vi "反控数据上传(子VI).vi"(8 "error in (no error)":errorcluster caption="错误输入（无错误）", 11 "QN":string) -> (0 "error out":errorcluster caption="错误输出")   [LabVIEW 2016, in "数据传输系统.lvlib"]
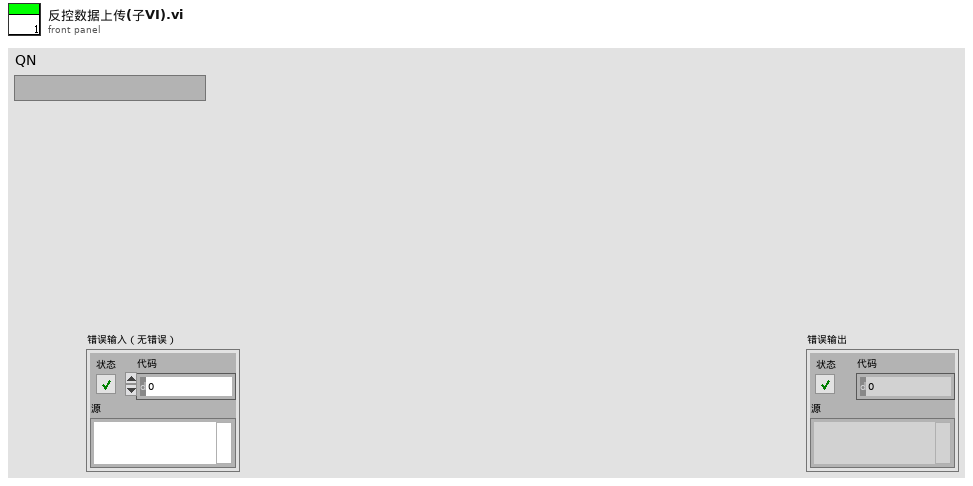
[diagram p1: front panel]
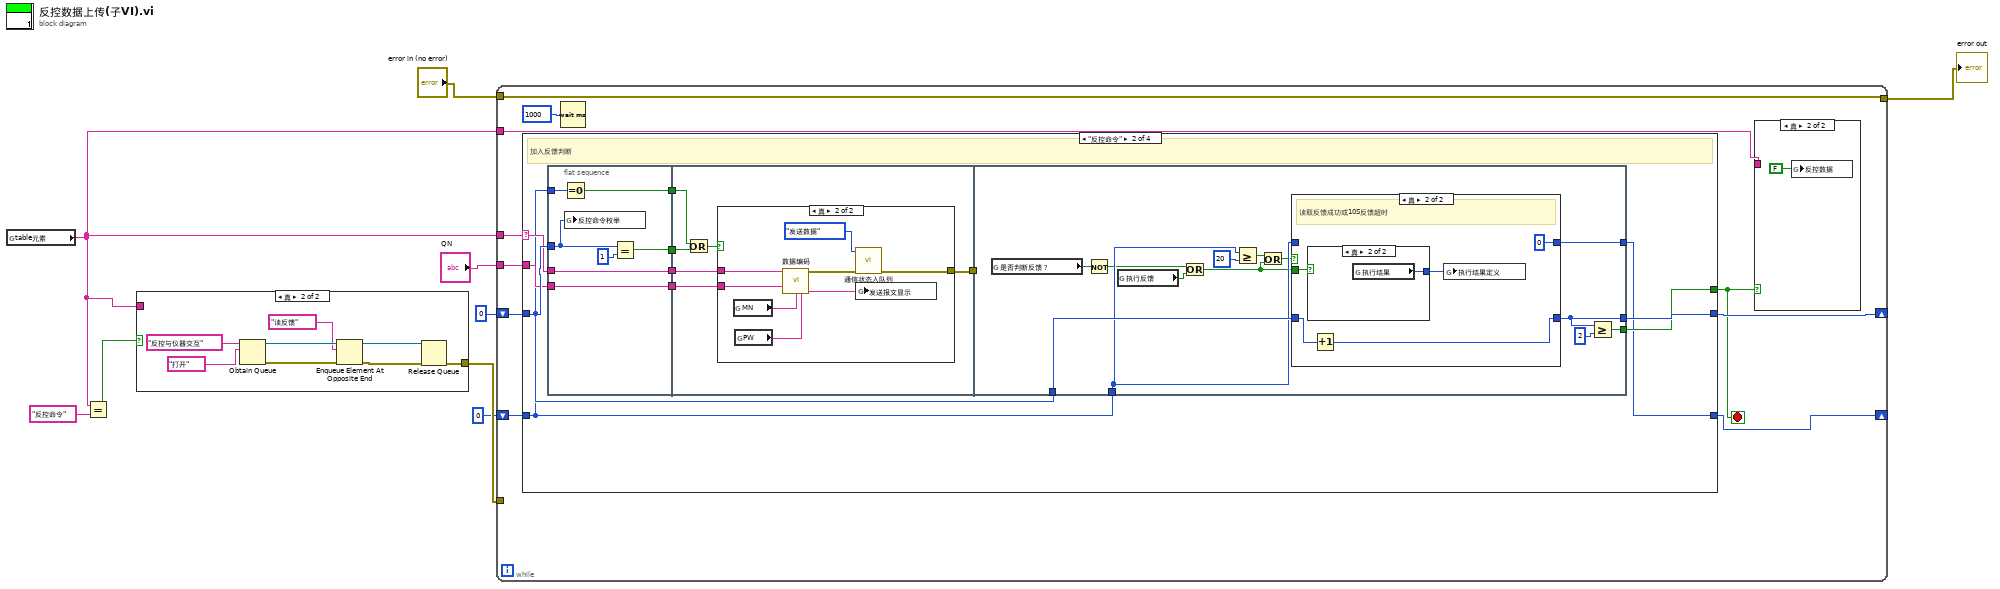
[diagram p0: block diagram]
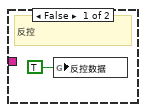
[diagram p3: hidden frame]
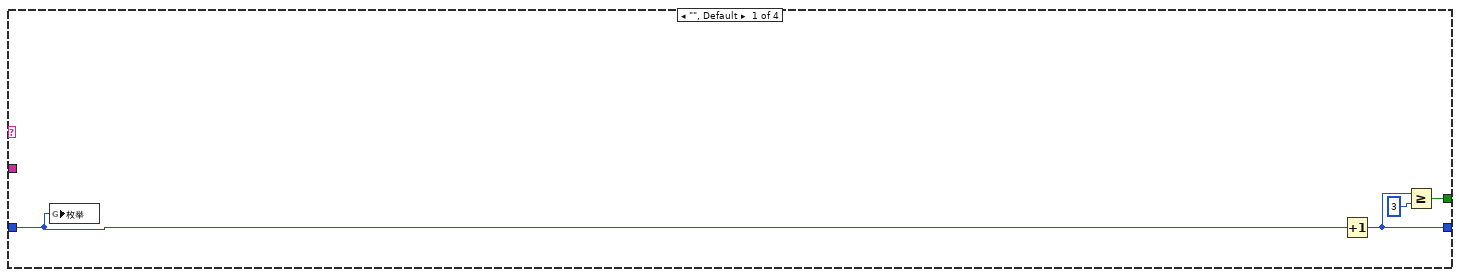
[diagram p4: hidden frame]
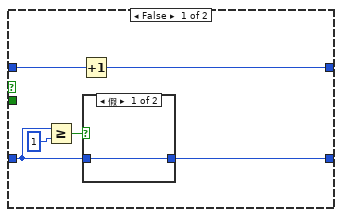
[diagram p6: hidden frame]
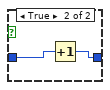
[diagram p7: hidden frame]
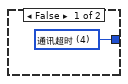
[diagram p8: hidden frame]
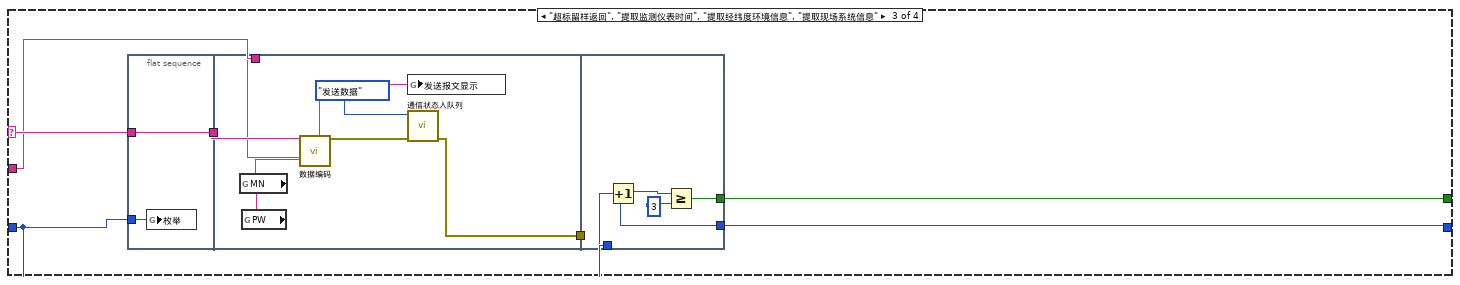
[diagram p9: hidden frame]
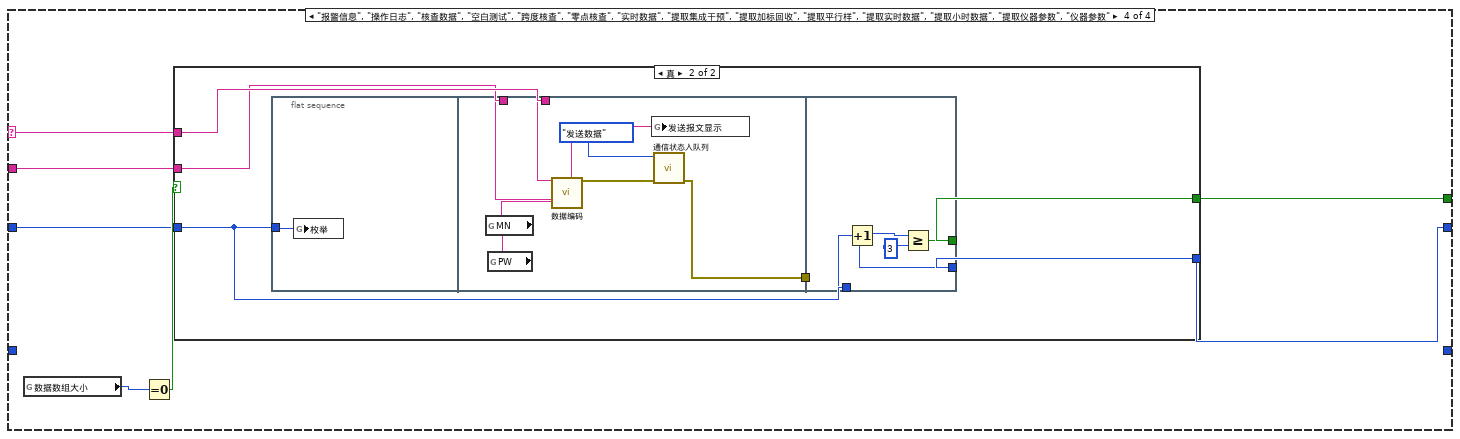
[diagram p10: hidden frame]
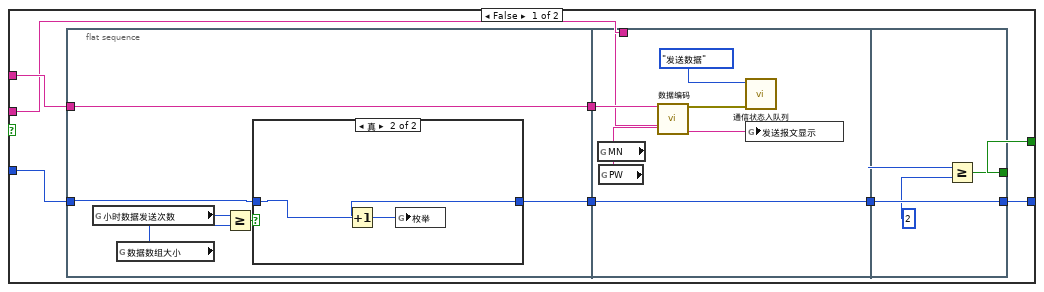
[diagram p11: hidden frame]
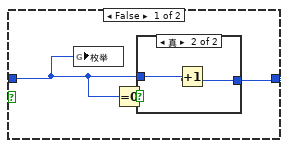
[diagram p12: hidden frame]
diagram:
  n1 = global read "全局1.vi" "table元素"() -> (w2:string)
  n2 = Equal?(x=w2, y="反控命令") -> (x = y?=w1:bool)
  n3 = case shown="真" w1 {
    tunnel: [_ w10] -> w5
    tunnel: w2 -> [_ _]
    frame False {
    }
    frame True {
      n4 = Obtain Queue(name (unnamed)="反控与仪器交互" ("名称（未命名）"), element data type="打开" ("读取写入选择")) -> (queue out=w15:refnum<queue>, error out=w14:errorcluster)  [unwired: 3 in, 1 out]
      n5 = Enqueue Element At Opposite End(queue=w15, element="读反馈" ("读取写入选择"), error in (no error)=w14) -> (queue out=w12:refnum<queue>, error out=w11:errorcluster)  [unwired: 1 in, 1 out]
      n6 = Release Queue(queue=w12, error in (no error)=w11) -> (error out=w10:errorcluster)  [unwired: 1 in, 2 out]
    }
  }
  n7 = while {
    tunnel: w2 -> [w27]
    shift-right: [w25] -> _
    shift-left: 0 -> [w26]
    tunnel: w2 -> [w23]
    tunnel: "QN" -> [w21]
    tunnel: "error in (no error)" -> [w20]
    tunnel: [w20] -> w6
    tunnel: w5 -> [_]
    shift-right: [w18] -> _
    shift-left: 0 -> [w19]
    stop <- w24 stop-if-true
    n8 = case shown="\"反控命令\"" w27 {
      selector: w27 -> [_ w42 w102 w119]
      tunnel: w26 -> [w32 w43 w99 w118]
      tunnel: [w31 w40 w98 w123] -> w24
      tunnel: [w30 w41 w97 w122] -> w25
      tunnel: w21 -> [_ w39 w96 w117]
      tunnel: w19 -> [_ w35 _ _]
      tunnel: [_ w37 _ _] -> w18
      frame "", Default {
        n9 = global write "全局1.vi" "枚举"(w32) -> ()
        n10 = Increment(x=w32) -> (x+1=w30:i32)
        n11 = Greater Or Equal?(x=w30, y=3) -> (x >= y?=w31:bool)
      }
      frame "反控命令" {
        # "加入反馈判断"
        n12 = flat-sequence {
          tunnel: w42 -> [w52]
          tunnel: [w52] -> w45
          tunnel: w43 -> [w50]
          tunnel: w39 -> [w51]
          tunnel: [w51] -> w38
          tunnel: [w48] -> w36
          tunnel: w35 -> [w47]
          tunnel: [w46] -> w34
          tunnel: w45 -> [w58]
          tunnel: [w57] -> w44
          tunnel: w38 -> [w56]
          tunnel: w36 -> [w54]
          tunnel: w34 -> [w53]
          tunnel: w44 -> [_]
          tunnel: w43 -> [w78]
          tunnel: [w77] -> w40
          tunnel: [w76] -> w41
          tunnel: w35 -> [w74]
          tunnel: [w75] -> w37
          frame #0 {
            n13 = Equal To 0?(x=w47) -> (x = 0?=w46:bool)
            n14 = global write "全局 反控命令枚举.vi" "反控命令枚举"(w50) -> ()
            n15 = Equal?(x=w50, y=1) -> (x = y?=w48:bool)
          }
          frame #1 {
            n16 = Or(x=w53, y=w54) -> (x .or. y?=w55:bool)
            n17 = case shown="真" w55 {
              tunnel: w58 -> [_ w61]
              tunnel: [_ w60] -> w57
              tunnel: w56 -> [_ w59]
              frame False {
              }
              frame True {
                n18 = global read "断电保存全局.vi" "MN"() -> (w66:string)
                n19 = global read "断电保存全局.vi" "PW"() -> (w65:string)
                n20 = call "数据编码.vi"("table输入"=w61, "QN"=w59, "MN"=w66, "PW"=w65) -> ("错误常量"=w63:errorcluster, "通讯包字符串"=w64:string)  [unwired: 10 in]
                n21 = call "通信状态入队列.vi"("错误输入（无错误）"=w63, "枚举"=enum16{"打开连接", "发送数据", "读取数据", "数据处理", "关闭连接"}."发送数据") -> ("错误输出"=w60:errorcluster)  [unwired: 9 in]
                n22 = global write "全局1.vi" "发送报文显示"(w64) -> ()
              }
            }
          }
          frame #2 {
            n23 = global read "全局 反控命令枚举.vi" "是否判断反馈？"() -> (w69:bool)
            n24 = Not(x=w69) -> (.not. x?=w68:bool)
            n25 = global read "全局 反控命令枚举.vi" "执行反馈"() -> (w70:bool)
            n26 = Or(x=w68, y=w70) -> (x .or. y?=w67:bool)
            n27 = Greater Or Equal?(x=w74, y=20) -> (x >= y?=w71:bool)
            n28 = Or(x=w71, y=w67) -> (x .or. y?=w72:bool)
            n29 = case shown="真" w72 {
              tunnel: w78 -> [w81 w93]
              tunnel: [w80 w92] -> w76
              tunnel: w74 -> [w85 _]
              tunnel: [w84 0] -> w75
              tunnel: w67 -> [_ w91]
              frame False {
                n30 = Greater Or Equal?(x=w81, y=1) -> (x >= y?=w82:bool)
                n31 = Increment(x=w85) -> (x+1=w84:i32)
                n32 = case shown="假" w82 {
                  tunnel: w81 -> [w86 w88]
                  tunnel: [w86 w87] -> w80
                  frame False {
                  }
                  frame True {
                    n33 = Increment(x=w88) -> (x+1=w87:i32)
                  }
                }
              }
              frame True {
                # "读取反馈成功或10S反馈超时"
                n34 = case shown="真" w91 {
                  tunnel: [w94 w95] -> w90
                  frame False {
                    w94 = u16 4 items=["执行成功"=1, "执行失败，但不知道原因"=2, "命令请求条件错误"=3, "通讯超时"=4, "系统繁忙不能执行"=5, "系统故障"=6, "没有数据"=100] ("执行结果定义")
                  }
                  frame True {
                    n35 = global read "全局 反控命令枚举.vi" "执行结果"() -> (w95:u16)
                  }
                }
                n36 = Increment(x=w93) -> (x+1=w92:i32)
                n37 = global write "全局 反控命令枚举.vi" "执行结果定义"(w90) -> ()
              }
            }
            n38 = Greater Or Equal?(x=w76, y=2) -> (x >= y?=w77:bool)
          }
        }
      }
      frame "超标留样返回", "提取监测仪表时间", "提取经纬度环境信息", "提取现场系统信息" {
        n39 = flat-sequence {
          tunnel: w102 -> [w104]
          tunnel: [w104] -> w101
          tunnel: w99 -> [w103]
          tunnel: w101 -> [w107]
          tunnel: [w106] -> w100
          tunnel: w96 -> [w105]
          tunnel: w100 -> [_]
          tunnel: w99 -> [w115]
          tunnel: [w114] -> w98
          tunnel: [w113] -> w97
          frame #0 {
            n40 = global write "全局1.vi" "枚举"(w103) -> ()
          }
          frame #1 {
            n41 = global read "断电保存全局.vi" "MN"() -> (w112:string)
            n42 = global read "断电保存全局.vi" "PW"() -> (w111:string)
            n43 = call "数据编码.vi"("table输入"=w107, "QN"=w105, "MN"=w112, "PW"=w111) -> ("错误常量"=w109:errorcluster, "通讯包字符串"=w110:string)  [unwired: 10 in]
            n44 = global write "全局1.vi" "发送报文显示"(w110) -> ()
            n45 = call "通信状态入队列.vi"("错误输入（无错误）"=w109, "枚举"=enum16{"打开连接", "发送数据", "读取数据", "数据处理", "关闭连接"}."发送数据") -> ("错误输出"=w106:errorcluster)  [unwired: 9 in]
          }
          frame #2 {
            n46 = Increment(x=w115) -> (x+1=w113:i32)
            n47 = Greater Or Equal?(x=w113, y=3) -> (x >= y?=w114:bool)
          }
        }
      }
      frame "报警信息", "操作日志", "核查数据", "空白测试", "跨度核查", "零点核查", "实时数据", "提取集成干预", "提取加标回收", "提取平行样", "提取实时数据", "提取小时数据", "提取仪器参数", "仪器参数" {
        n48 = global read "全局 数据数组大小.vi" "数据数组大小"() -> (w121:i32)
        n49 = Equal To 0?(x=w121) -> (x = 0?=w120:bool)
        n50 = case shown="真" w120 {
          tunnel: [w128 w158] -> w123
          tunnel: [w127 w159] -> w122
          tunnel: w119 -> [w126 w161]
          tunnel: w118 -> [w125 w160]
          tunnel: w117 -> [w124 w157]
          frame False {
            n51 = flat-sequence {
              tunnel: w125 -> [w134]
              tunnel: [w132] -> w131
              tunnel: w126 -> [w133]
              tunnel: [w133] -> w130
              tunnel: w131 -> [w153]
              tunnel: [w153] -> w129
              tunnel: w130 -> [w147]
              tunnel: w124 -> [w146]
              tunnel: w129 -> [w156]
              tunnel: [w156] -> w127
              tunnel: [w155] -> w128
              frame #0 {
                n52 = global read "全局 小时数据发送次数.vi" "小时数据发送次数"() -> (w136:i32)
                n53 = global read "全局 数据数组大小.vi" "数据数组大小"() -> (w137:i32)
                n54 = Greater Or Equal?(x=w136, y=w137) -> (x >= y?=w135:bool)
                n55 = case shown="真" w135 {
                  tunnel: w134 -> [w139 w145]
                  tunnel: [w140 w144] -> w132
                  frame False {
                    n56 = global write "全局1.vi" "枚举"(w139) -> ()
                    n57 = Equal To 0?(x=w139) -> (x = 0?=w138:bool)
                    n58 = case shown="真" w138 {
                      tunnel: w139 -> [w141 w143]
                      tunnel: [w141 w142] -> w140
                      frame False {
                      }
                      frame True {
                        n59 = Increment(x=w143) -> (x+1=w142:i32)
                      }
                    }
                  }
                  frame True {
                    n60 = Increment(x=w145) -> (x+1=w144:i32)
                    n61 = global write "全局1.vi" "枚举"(w144) -> ()
                  }
                }
              }
              frame #1 {
                n62 = global read "断电保存全局.vi" "MN"() -> (w148:string)
                n63 = global read "断电保存全局.vi" "PW"() -> (w149:string)
                n64 = call "数据编码.vi"("table输入"=w147, "QN"=w146, "MN"=w148, "PW"=w149) -> ("错误常量"=w151:errorcluster, "通讯包字符串"=w150:string)  [unwired: 10 in]
                n65 = call "通信状态入队列.vi"("错误输入（无错误）"=w151, "枚举"=enum16{"打开连接", "发送数据", "读取数据", "数据处理", "关闭连接"}."发送数据") -> ()  [unwired: 9 in, 1 out]
                n66 = global write "全局1.vi" "发送报文显示"(w150) -> ()
              }
              frame #2 {
                n67 = Greater Or Equal?(x=w156, y=2) -> (x >= y?=w155:bool)
              }
            }
          }
          frame True {
            n68 = flat-sequence {
              tunnel: w160 -> [w163]
              tunnel: [w166] -> w162
              tunnel: w161 -> [w165]
              tunnel: w157 -> [w164]
              tunnel: w162 -> [_]
              tunnel: [w174] -> w158
              tunnel: [w173] -> w159
              tunnel: w160 -> [w172]
              frame #0 {
                n69 = global write "全局1.vi" "枚举"(w163) -> ()
              }
              frame #1 {
                n70 = global read "断电保存全局.vi" "MN"() -> (w171:string)
                n71 = global read "断电保存全局.vi" "PW"() -> (w170:string)
                n72 = call "数据编码.vi"("table输入"=w165, "QN"=w164, "MN"=w171, "PW"=w170) -> ("错误常量"=w168:errorcluster, "通讯包字符串"=w169:string)  [unwired: 10 in]
                n73 = global write "全局1.vi" "发送报文显示"(w169) -> ()
                n74 = call "通信状态入队列.vi"("错误输入（无错误）"=w168, "枚举"=enum16{"打开连接", "发送数据", "读取数据", "数据处理", "关闭连接"}."发送数据") -> ("错误输出"=w166:errorcluster)  [unwired: 9 in]
              }
              frame #2 {
                n75 = Increment(x=w172) -> (x+1=w173:i32)
                n76 = Greater Or Equal?(x=w173, y=3) -> (x >= y?=w174:bool)
              }
            }
          }
        }
      }
    }
    n77 = Wait (ms)(milliseconds to wait=u32 1000 ("等待时间（毫秒）")) -> ()  [unwired: 1 out]
    n78 = case shown="真" w24 {
      tunnel: w23 -> [_ _]
      frame False {
        # "反控"
        n79 = global write "全局1.vi" "反控数据"(TRUE ("反控数据")) -> ()
      }
      frame True {
        n80 = global write "全局1.vi" "反控数据"(FALSE ("反控数据")) -> ()
      }
    }
  }
  "error out" <- w6
